vi "LJT7I2C_RangeFinder.vi"(4 "Scan Period":dbl format="%.2f", 5 "Previous Scan Value":dbl format="%.2f", 6 "Present scan array":dbl[](array[numeric]) format="%.2f", 7 "Value to Output":dbl format="%.2f", 8 "Ch Description":T1={"Ch Name"="", "Type"="", "Function"=enum."Analogue Input", "Ch State"=enum."On", "Calibration type"=enum."Raw", "A"=2.0, "B"=3.0, "C"=224.0, "D"=5.0, "Comments"="", "Address"={"Main"=502, "Ch."=0, "Sub"=0, "Port Name"="192.168.124.53"}, "String"="", "Duty"=65535} {"Duty" format="%.0b"; "D" format="%#_5g"; "C" format="%#_5g"; "B" format="%#_5g"; "A" format="%#_5g"}, 9 "Ch names":string[](array[string])) -> (0 "Scan comment":string, 1 "Output":dbl=101.0 format="%.7f")   [LabVIEW 2015]
uses:
  ADAM Client/Sub VIs/ADAM Controls/Ch_description_ADAM.ctl
  ADAM Client/Sub VIs/ADAM Controls/Module_type_ADAM.ctl
  ADAM Client/Sub VIs/ADAM Controls/Function_ADAM.ctl
  ADAM Client/Sub VIs/ADAM Controls/Channel_State.ctl
  ADAM Client/Sub VIs/ADAM Controls/Calib_type_ADAM.ctl
  ADAM Client/Sub VIs/ADAM Controls/Address.ctl
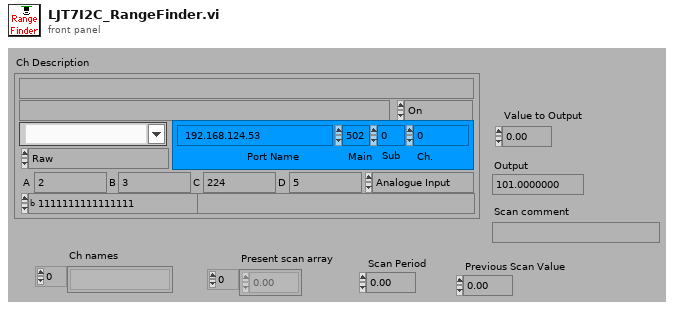
[diagram p1: front panel]
types:
  T1 = typedef "Ch_description_ADAM.ctl" = cluster{"Ch Name":string, "Type":T2, "Function":T3, "Ch State":T4, "Calibration type":T5, "A":dbl, "B":dbl, "C":dbl, "D":dbl, "Comments":string, "Address":T6, "String":string, "Duty":u16}
  T2 = typedef "Module_type_ADAM.ctl" = string
  T3 = typedef "Function_ADAM.ctl" = enum16{"Analogue Input", "Digital Input", "Event counter", "Event rate", "Analogue Output", "Digital Output", "Relay Output"}
  T4 = typedef "Channel_State.ctl" = enum16{"On", "Off", "Always On", "Always Off"}
  T5 = typedef "Calib_type_ADAM.ctl" = enum16{"Raw", "Bx + A", "Cx^2 + Bx + A", "Dx^3 + Cx^2 + Bx + A", "In Band", "Hi-Tec Q", "Hi-Tec M_dot", "Text"}
  T6 = typedef "Address.ctl" = cluster{"Main":i32, "Ch.":i32, "Sub":i32, "Port Name":string}
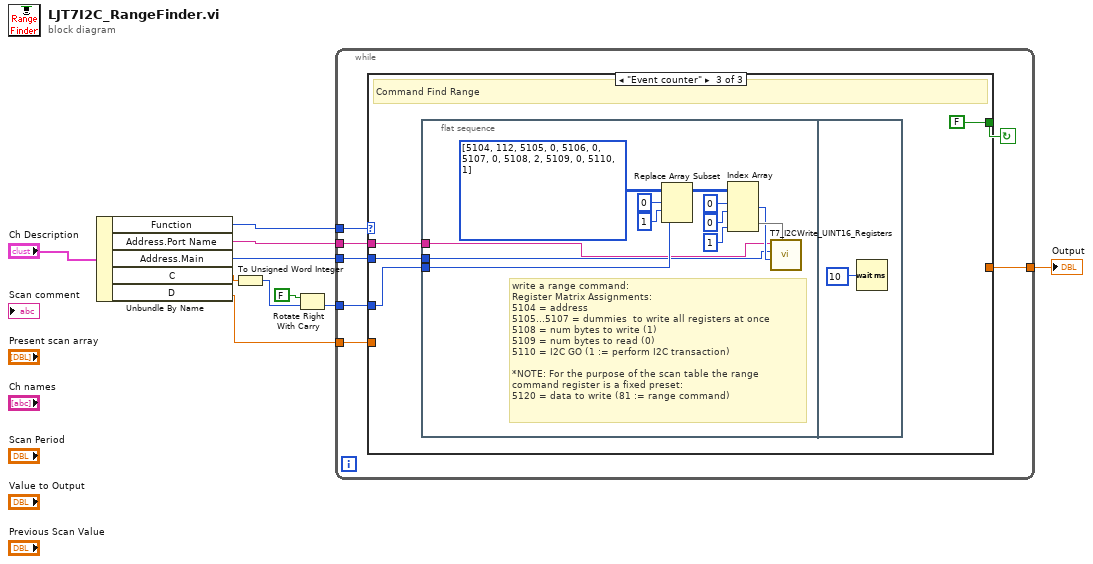
[diagram p0: block diagram]
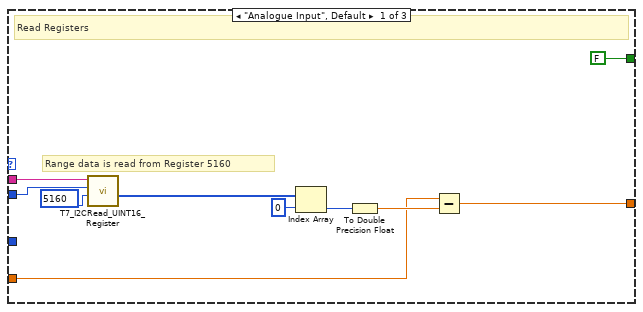
[diagram p2: hidden frame]
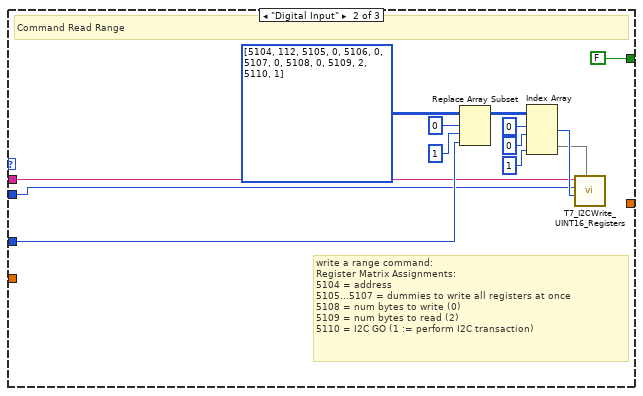
[diagram p3: hidden frame]
diagram:
  n1 = Unbundle By Name("Ch Description") -> ("Function"=w9:T3, "Address.Port Name"=w4:string, "Address.Main"=w3:i32, "C"=w2:dbl, "D"=w1:dbl)
  n2 = To Unsigned Word Integer(number=w2) -> (unsigned 16bit integer=w6:u16)
  n3 = Rotate Right With Carry(2:w6, 3:FALSE ("carry")) -> (0:w7:u16)  [unwired: 1 out]
  n4 = while {
    tunnel: w9 -> [w17]
    tunnel: [w15] -> w10
    tunnel: w7 -> [w14]
    tunnel: w4 -> [w13]
    tunnel: w3 -> [w12]
    tunnel: w1 -> [w11]
    stop <- w16 continue-if-true
    n5 = case shown="\"Event counter\"" w17 {
      tunnel: [FALSE FALSE FALSE] -> w16
      tunnel: [w18 _ _] -> w15
      tunnel: w14 -> [_ w31 w43]
      tunnel: w13 -> [w22 w29 w42]
      tunnel: w12 -> [w21 w28 w41]
      tunnel: w11 -> [w19 _ _]
      frame "Analogue Input", Default {
        # "Range data is read from Register 5160"
        # "Read Registers"
        n6 = call "T7_I2CRead_UINT16_Register.vi"("FirstChannel"=5160, "Remote Port"=w21, "Remote IP Address"=w22) -> ("Raw Data Read"=w25:u16[])  [unwired: 6 in, 2 out]
        n7 = Index Array(array=w25, index=0) -> (element=w23:u16)
        n8 = To Double Precision Float(number=w23) -> (double precision float=w20:dbl)
        n9 = Subtract(x=w19, y=w20) -> (x-y=w18:dbl)
      }
      frame "Digital Input" {
        # "write a range command:\nRegister Matrix Assignments:\n5104 = address\n5105...5107 = dummies to write all registers at once\n5108 = num bytes to write (0)\n5109 = num bytes to read (2)\n5110 = I2C GO (1 := perform I2C transaction)"
        # "Command Read Range"
        n10 = Replace Array Subset(array=i32[][] [[5104, 112], [5105, 0], [5106, 0], [5107, 0], [5108, 0], [5109, 2], [5110, 1]], new element=w31, index (row)=0, index (col)=1 ("disabled index (col)")) -> (w30:i32[][])
        n11 = Index Array(array=w30, index (row) #1=0 ("disabled index (row)"), index (col) #1=0 ("disabled index (col)"), index (col) #2=1 ("index (col)")) -> (element #1=w36:i32, element #2=w35:i32[])  [unwired: 1 in]
        n12 = call "T7_I2CWrite_UINT16_Registers.vi"("Remote IP Address"=w29, "Remote Port"=w28, "Starting Address"=w36, "UINT16 to Write"=w35) -> ()  [unwired: 5 in, 2 out]
      }
      frame "Event counter" {
        # "Command Find Range"
        n13 = flat-sequence {
          tunnel: w43 -> [w48]
          tunnel: w42 -> [w46]
          tunnel: w41 -> [w45]
          frame #0 {
            # "write a range command:\nRegister Matrix Assignments:\n5104 = address\n5105...5107 = dummies  to write all registers at once\n5108 = num bytes to write (1)\n5109 = num bytes to read (0)\n5110 = I2C GO (1 := perform I2C transaction)\n\n*NOTE: For the purpose of the scan table the range\ncommand register is a fixed preset:\n5120 = data to write (81 := range command)"
            n14 = Replace Array Subset(array=i32[][] [[5104, 112], [5105, 0], [5106, 0], [5107, 0], [5108, 2], [5109, 0], [5110, 1]], new element=w48, index (row)=0, index (col)=1 ("disabled index (col)")) -> (w47:i32[][])
            n15 = Index Array(array=w47, index (row) #1=0 ("disabled index (row)"), index (col) #1=0 ("disabled index (col)"), index (col) #2=1 ("index (col)")) -> (element #1=w52:i32, element #2=w53:i32[])  [unwired: 1 in]
            n16 = call "T7_I2CWrite_UINT16_Registers.vi"("Remote IP Address"=w46, "Remote Port"=w45, "Starting Address"=w52, "UINT16 to Write"=w53) -> ()  [unwired: 5 in, 2 out]
          }
          frame #1 {
            n17 = Wait (ms)(milliseconds to wait=u32 10) -> ()  [unwired: 1 out]
          }
        }
      }
    }
  }
  "Output" <- w10
